vi "Get SDK Version.vi"(8 "error in (no error)":errorcluster) -> (0 "error out":errorcluster, 1 "Build":u8, 2 "Minor":u8, 3 "Major":u8)   [LabVIEW 2025, in "Logitech Devices.lvlib"]
uses:
  Logitech Devices.lvlib
  <vilib>/Utility/error.llb/Error Cluster From Error Code.vi
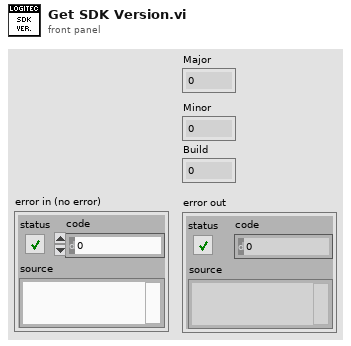
[diagram p1: front panel]
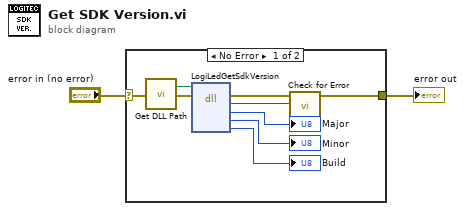
[diagram p0: block diagram]
diagram:
  n1 = case shown="No Error" "error in (no error)" {
    selector: "error in (no error)" -> [w6 w11]
    tunnel: [w10 w11] -> w1
    frame No Error {
      n2 = call "Get DLL Path.vi"() -> ("LG Hub SDK DLL"=w3:path)  [unwired: 3 in]
      n3 = dll-call lib="C:/Program Files/LGHUB/sdks/sdk_legacy_led_x86.dll" fn="LogiLedGetSdkVersion"(path in=w3, error in=w6) -> (error out=w5:errorcluster, "return type"=w4:u8, "majorNum"=→"Major":u8, "minorNum"=→"Minor":u8, "buildNum"=→"Build":u8)  [unwired: 4 in, 1 out]
      n4 = call "Check for Error.vi"("DLL-call return value"=w4, "error in (no error)"=w5) -> ("error out"=w10:errorcluster)  [unwired: 9 in]
    }
    frame Error {
    }
  }
  "error out" <- w1
